vi "Logger_Log_Data.vi"(8 "Data":dbl, 9 "Channel":string, 10 "Group":string, 11 "TDMS DevRef":T1) -> (0 "error out":errorcluster)   [LabVIEW 2017]
uses:
  <userlib>/836-Library/System/TDMS_V2/Support/TDMS_DevRef.ctl
  <userlib>/836-Library/System/TDMS_V2/Support/Logging_Settings.ctl
  <userlib>/836-Library/System/TDMS_V2/Support/Group_FIFO_Config.ctl
  <userlib>/836-Library/System/TDMS_V2/Support/Channel_FIFO_Config.ctl
  <vilib>/ErrorRing/Error Ring.xnode
panel:
  in  "Re-Search TDMS Info":bool
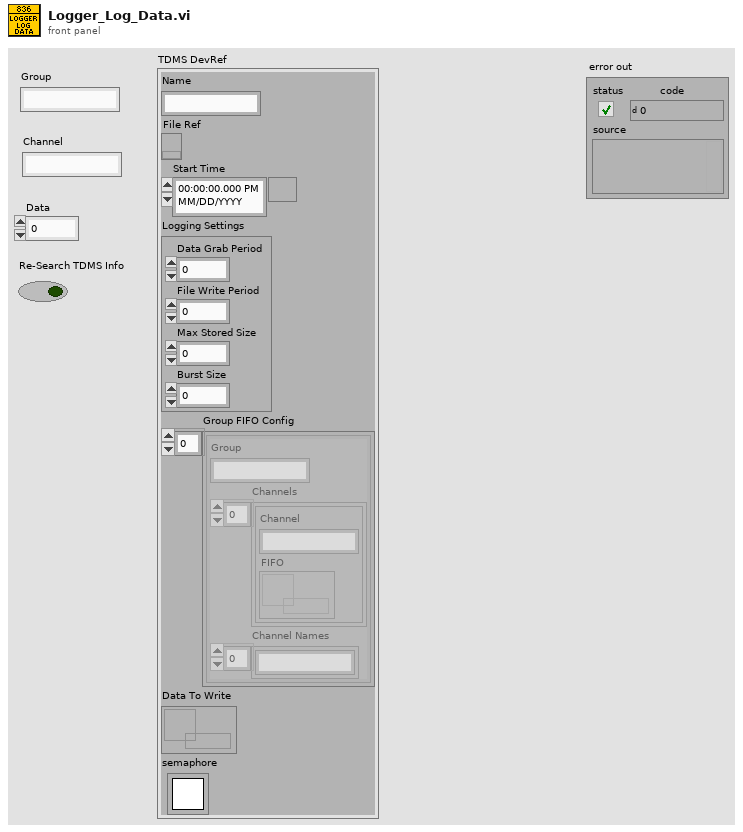
[diagram p1: front panel]
types:
  T1 = typedef "TDMS_DevRef.ctl" = cluster{"Name":string, "File Ref":refnum<k34>, "Start Time":timestamp, "Logging Settings":T2, "Group FIFO Config":T3[], "Data To Write":refnum<data-value>, "semaphore":T5}
  T2 = typedef "Logging_Settings.ctl" = cluster{"Data Grab Period":dbl, "File Write Period":dbl, "Max Stored Size":dbl, "Burst Size":dbl}
  T3 = typedef "Group_FIFO_Config.ctl" = cluster{"Group":string, "Channels":T4[], "Channel Names":string[]}
  T4 = typedef "Channel_FIFO_Config.ctl" = cluster{"Channel":string, "FIFO":refnum<k33>}
  T5 = typedef "Semaphore RefNum" = refnum<k1>
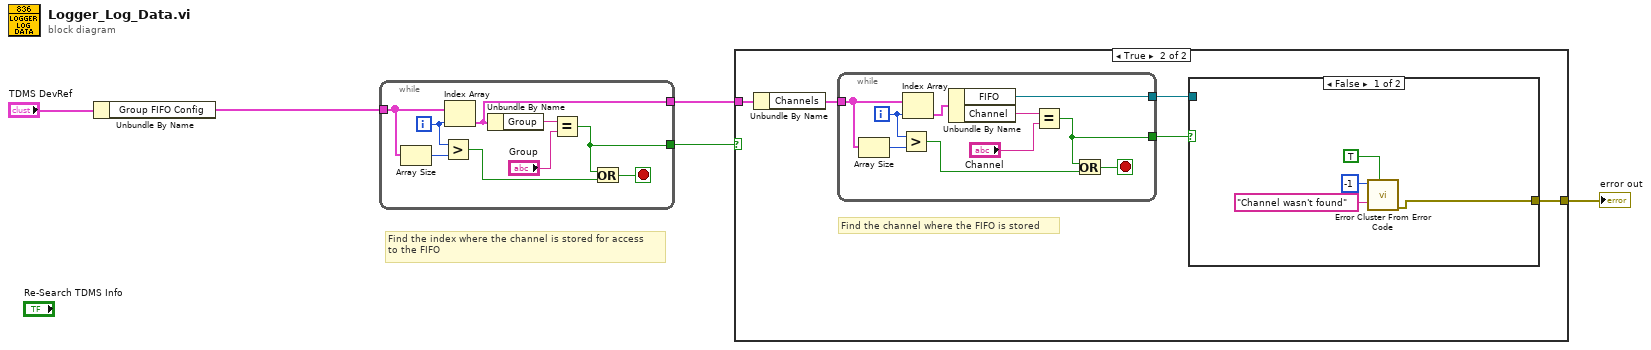
[diagram p0: block diagram]
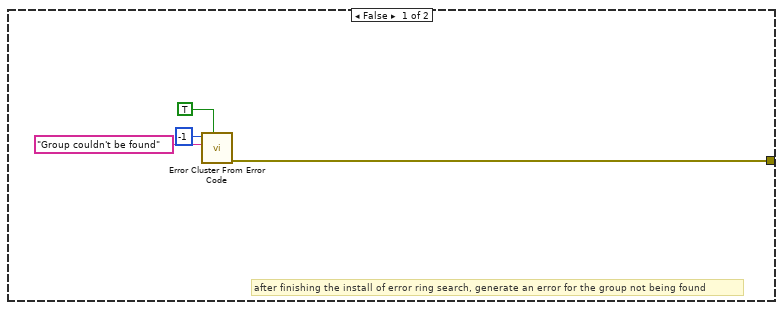
[diagram p2: hidden frame]
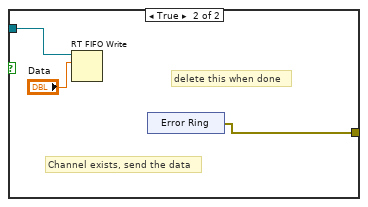
[diagram p3: hidden frame]
diagram:
  # "Find the index where the channel is stored for access\nto the FIFO"
  n1 = Unbundle By Name("TDMS DevRef") -> ("Group FIFO Config"=w4:T3[])
  n2 = while {
    tunnel: w4 -> [w10]
    tunnel: [w7] -> w3
    tunnel: [w6] -> w2
    i -> [w11]
    stop <- w12 stop-if-true
    n3 = Array Size(array=w10) -> (size(s)=w9:i32)
    n4 = Greater?(x=w11, y=w9) -> (0:w8:bool)
    n5 = Index Array(array=w10, index=w11) -> (element=w6:T3)
    n6 = Unbundle By Name(w6) -> ("Group"=w14:string)
    n7 = Equal?(x=w14, y="Group") -> (x = y?=w7:bool)
    n8 = Or(x=w7, y=w8) -> (x .or. y?=w12:bool)
  }
  n9 = case shown="True" w3 {
    tunnel: w2 -> [_ w23]
    tunnel: [w18 w19] -> w1
    frame False {
      # "after finishing the install of error ring search, generate an error for the group not being found"
      n10 = call <vilib>:"Error Cluster From Error Code.vi"("show call chain? (False)"=TRUE, "error message (\"\")"="Group couldn't be found" ("error message (\"\")"), "error code (0)"=-1) -> ("error out"=w18:errorcluster)  [unwired: 6 in]
    }
    frame True {
      # "Find the channel where the FIFO is stored"
      n11 = Unbundle By Name(w23) -> ("Channels"=w22:T4[])
      n12 = while {
        tunnel: w22 -> [w37]
        tunnel: [w34] -> w21
        tunnel: [w32] -> w20
        i -> [w38]
        stop <- w39 stop-if-true
        n13 = Array Size(array=w37) -> (size(s)=w36:i32)
        n14 = Greater?(x=w38, y=w36) -> (0:w35:bool)
        n15 = Index Array(array=w37, index=w38) -> (element=w41:T4)
        n16 = Unbundle By Name(w41) -> ("FIFO"=w32:refnum<k33>, "Channel"=w40:string)
        n17 = Equal?(x=w40, y="Channel") -> (x = y?=w34:bool)
        n18 = Or(x=w34, y=w35) -> (x .or. y?=w39:bool)
      }
      n19 = case shown="False" w21 {
        tunnel: w20 -> [_ w30]
        tunnel: [w24 w28] -> w19
        frame False {
          n20 = call <vilib>:"Error Cluster From Error Code.vi"("show call chain? (False)"=TRUE, "error message (\"\")"="Channel wasn't found" ("error message (\"\")"), "error code (0)"=-1) -> ("error out"=w24:errorcluster)  [unwired: 6 in]
        }
        frame True {
          # "delete this when done"
          # "Channel exists, send the data"
          n21 = RT FIFO Write(0:w30, 1:"Data") -> ()  [unwired: 3 in, 4 out]
          n22 = xnode "Error Ring"() -> ("error out"=w28:errorcluster)
        }
      }
    }
  }
  "error out" <- w1
